vi "Generate_Vertex_Array.vi"(4 "Sensor Z":dbl[][](array[numeric]), 5 "Z Baseline":dbl[][](array[numeric]), 6 "Sensor Y":dbl[][](array[numeric]), 7 "Y Baseline":dbl[][](array[numeric]), 8 "Sensor X":dbl[][](array[numeric]), 9 "Size":i32[](array[numeric]), 10 "Gain":dbl[](array[numeric]), 11 "X Baseline":dbl[][](array[numeric])) -> (3 "Init Vertex Array":cluster{"x":dbl, "y":dbl, "z":dbl}[](array[cluster]))   [LabVIEW 2018]
uses:
  <vilib>/Native 3D Graph/xcontrol/3DPC_SurfacePlot.xctl
panel:
  out "3D Graph":refnum<class "Base Datatype.lvclass">[](xcontrol)
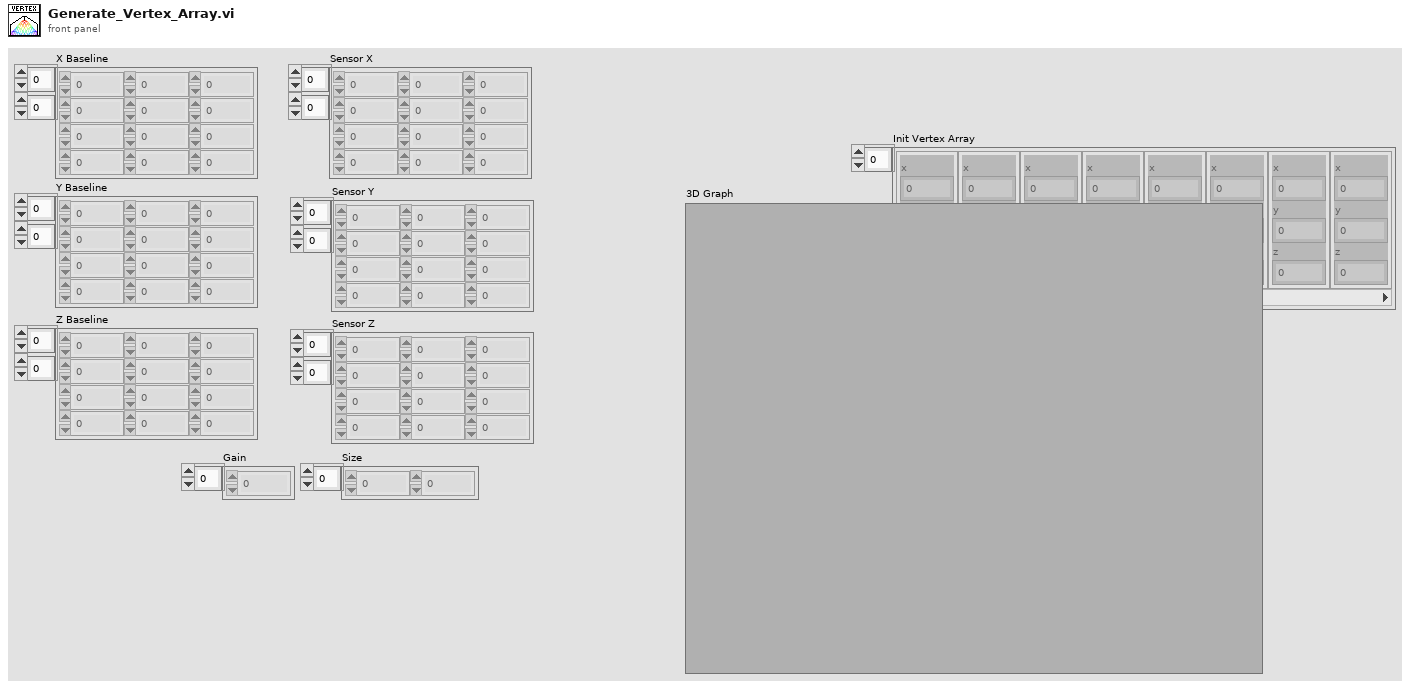
[diagram p1: front panel]
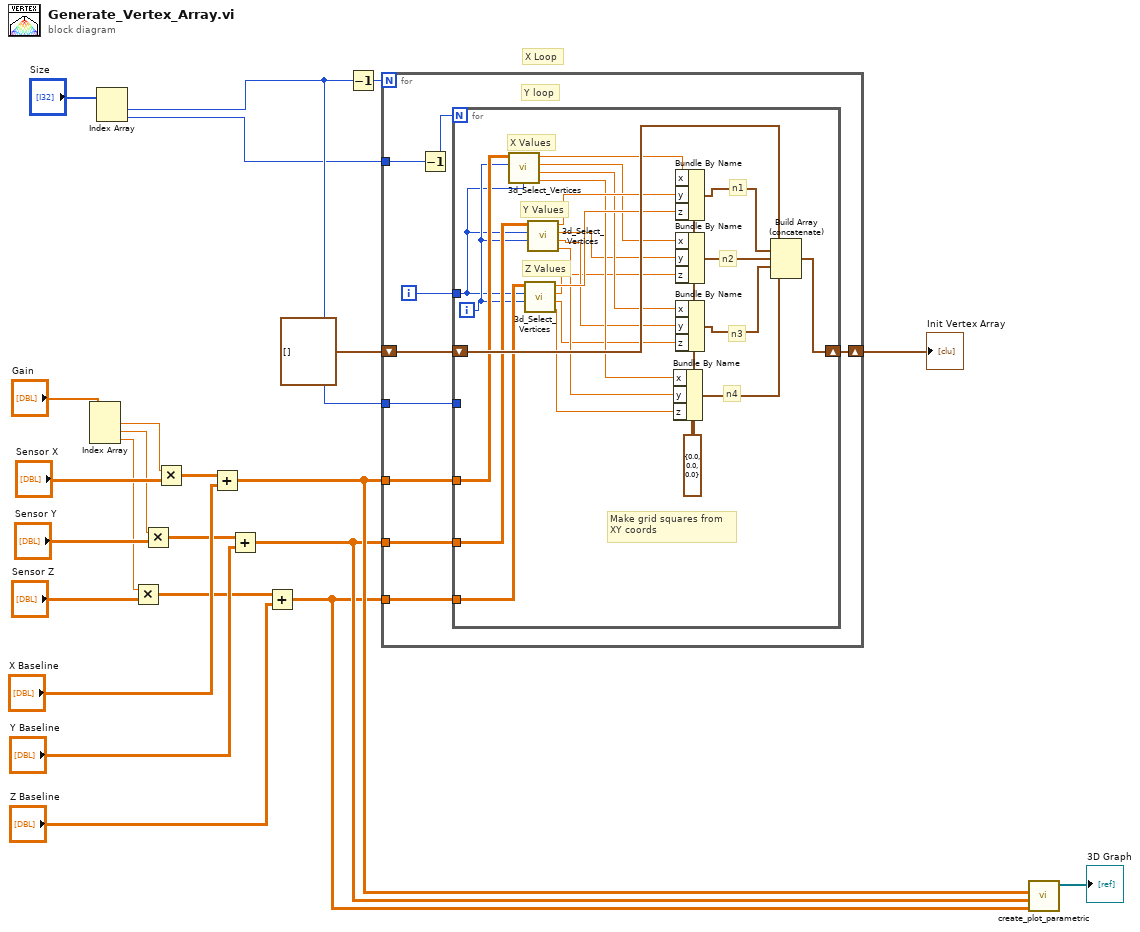
[diagram p0: block diagram]
diagram:
  # "X Loop"
  n1 = Index Array(array="Gain") -> (element #1=w19:dbl, element #2=w17:dbl, element #3=w15:dbl)  [unwired: 3 in]
  n2 = Index Array(array="Size") -> (element #1=w6:i32, element #2=w5:i32)  [unwired: 2 in]
  n3 = Multiply(x=w15, y="Sensor Z") -> (x*y=w9:dbl[][])
  n4 = Multiply(x=w17, y="Sensor Y") -> (x*y=w11:dbl[][])
  n5 = Multiply(x=w19, y="Sensor X") -> (x*y=w12:dbl[][])
  n6 = Add(x=w12, y="X Baseline") -> (x+y=w3:dbl[][])
  n7 = Add(x=w11, y="Y Baseline") -> (x+y=w2:dbl[][])
  n8 = Add(x=w9, y="Z Baseline") -> (x+y=w1:dbl[][])
  n9 = Decrement(x=w6) -> (x-1=w22:i32)
  n10 = for {
    N: w22 -> [_]
    shift-right: [w30] -> w21
    shift-left: cluster{"x":dbl, "y":dbl, "z":dbl}[] [] ("Vertex Array") -> [w31]
    tunnel: w6 -> [w28]
    tunnel: w5 -> [w27]
    tunnel: w3 -> [w26]
    tunnel: w2 -> [w25]
    tunnel: w1 -> [w24]
    i -> [w29]
    # "Y loop"
    n11 = Decrement(x=w27) -> (x-1=w32:i32)
    n12 = for {
      N: w32 -> [_]
      tunnel: w29 -> [w46]
      shift-right: [w50] -> w30
      shift-left: w31 -> [w56]
      tunnel: w28 -> [_]
      tunnel: w26 -> [w55]
      tunnel: w25 -> [w49]
      tunnel: w24 -> [w48]
      i -> [w47]
      w39 = cluster{"x":dbl, "y":dbl, "z":dbl} {"x"=0.0, "y"=0.0, "z"=0.0} ("3D Point")
      # "n4"
      # "n3"
      # "n2"
      # "n1"
      # "Z Values"
      # "Y Values"
      # "X Values"
      # "Make grid squares from\nXY coords"
      n13 = call "3d_Select_Vertices.vi"("Y index"=w46, "X index"=w47, "GRID Array"=w55) -> ("V4"=w40:dbl, "V3"=w41:dbl, "V2"=w42:dbl, "V1"=w45:dbl)  [unwired: 5 in]
      n14 = call "3d_Select_Vertices.vi"("Y index"=w47, "X index"=w46, "GRID Array"=w48) -> ("V4"=w33:dbl, "V3"=w34:dbl, "V2"=w35:dbl, "V1"=w43:dbl)  [unwired: 5 in]
      n15 = call "3d_Select_Vertices.vi"("Y index"=w47, "X index"=w46, "GRID Array"=w49) -> ("V4"=w36:dbl, "V3"=w37:dbl, "V2"=w38:dbl, "V1"=w44:dbl)  [unwired: 5 in]
      n16 = Bundle By Name(cluster=w39, "x"=w40, "y"=w36, "z"=w33) -> (w51:cluster{"x":dbl, "y":dbl, "z":dbl})
      n17 = Bundle By Name(cluster=w39, "x"=w45, "y"=w44, "z"=w43) -> (w54:cluster{"x":dbl, "y":dbl, "z":dbl})
      n18 = Bundle By Name(cluster=w39, "x"=w42, "y"=w38, "z"=w35) -> (w53:cluster{"x":dbl, "y":dbl, "z":dbl})
      n19 = Bundle By Name(cluster=w39, "x"=w41, "y"=w37, "z"=w34) -> (w52:cluster{"x":dbl, "y":dbl, "z":dbl})
      n20 = Build Array (concatenate)(w56, w54, w53, w52, w51) -> (w50:cluster{"x":dbl, "y":dbl, "z":dbl}[])
    }
  }
  "Init Vertex Array" <- w21
  n21 = call <vilib>:"create_plot_parametric.vi"("z matrix"=w1, "y matrix"=w2, "x matrix"=w3) -> ("plots out"=→"3D Graph":refnum<class "Base Datatype.lvclass">[])  [unwired: 2 in, 6 out]
